vi "Base marwan_eleve.vi"() -> ()   [LabVIEW 2018]
uses:
  Global Humdidtiy 4.vi
  Global temperateurvi.vi
  Global  pressure.vi
  <vilib>/Instr/_visa.llb/VISA Configure Serial Port (Instr).vi
  <vilib>/express/express arith-compare/Formula/XNode/ExpressFormulaBlockNode.xnode
panel:
  out "Waveform Humidity 2":dbl(graph)
  out "Waveform Pressure 2":dbl(graph)
  out "Waveform temperateur  2":dbl(graph)
  out "Humidity 2":dbl
  out "Pressure 2":dbl
  out "Temperateur 2":dbl
  out "Chaîne 2":string
  out "Kelvin":dbl
  out "Fahrenheit":dbl
  in  "Pause":bool
  out "Moyen":dbl
  out "Moyen":dbl
  out "Moyen":dbl
  out "MAX":dbl
  out "MIN":dbl
  out "MIN":dbl
  out "MAX":dbl
  out "MIN":dbl
  out "MAX":dbl
  out "Waveform Humidity":dbl(graph)
  out "Waveform Pressure":dbl(graph)
  out "Waveform temperateur":dbl(graph)
  out "Humidity":dbl
  out "Pressure":dbl
  out "Temperateur":dbl
  out "Chaîne":string
  in  "stop":bool
  in  "Nom de ressource VISA":refnum<visa-resource-name>
  # "1. Brancher la carte Arduino sur un port USB\n2. Choisir le port COM de la carte dans la liste déroulante \"Nom de ressource VISA\"\n3. Lancer le programme"
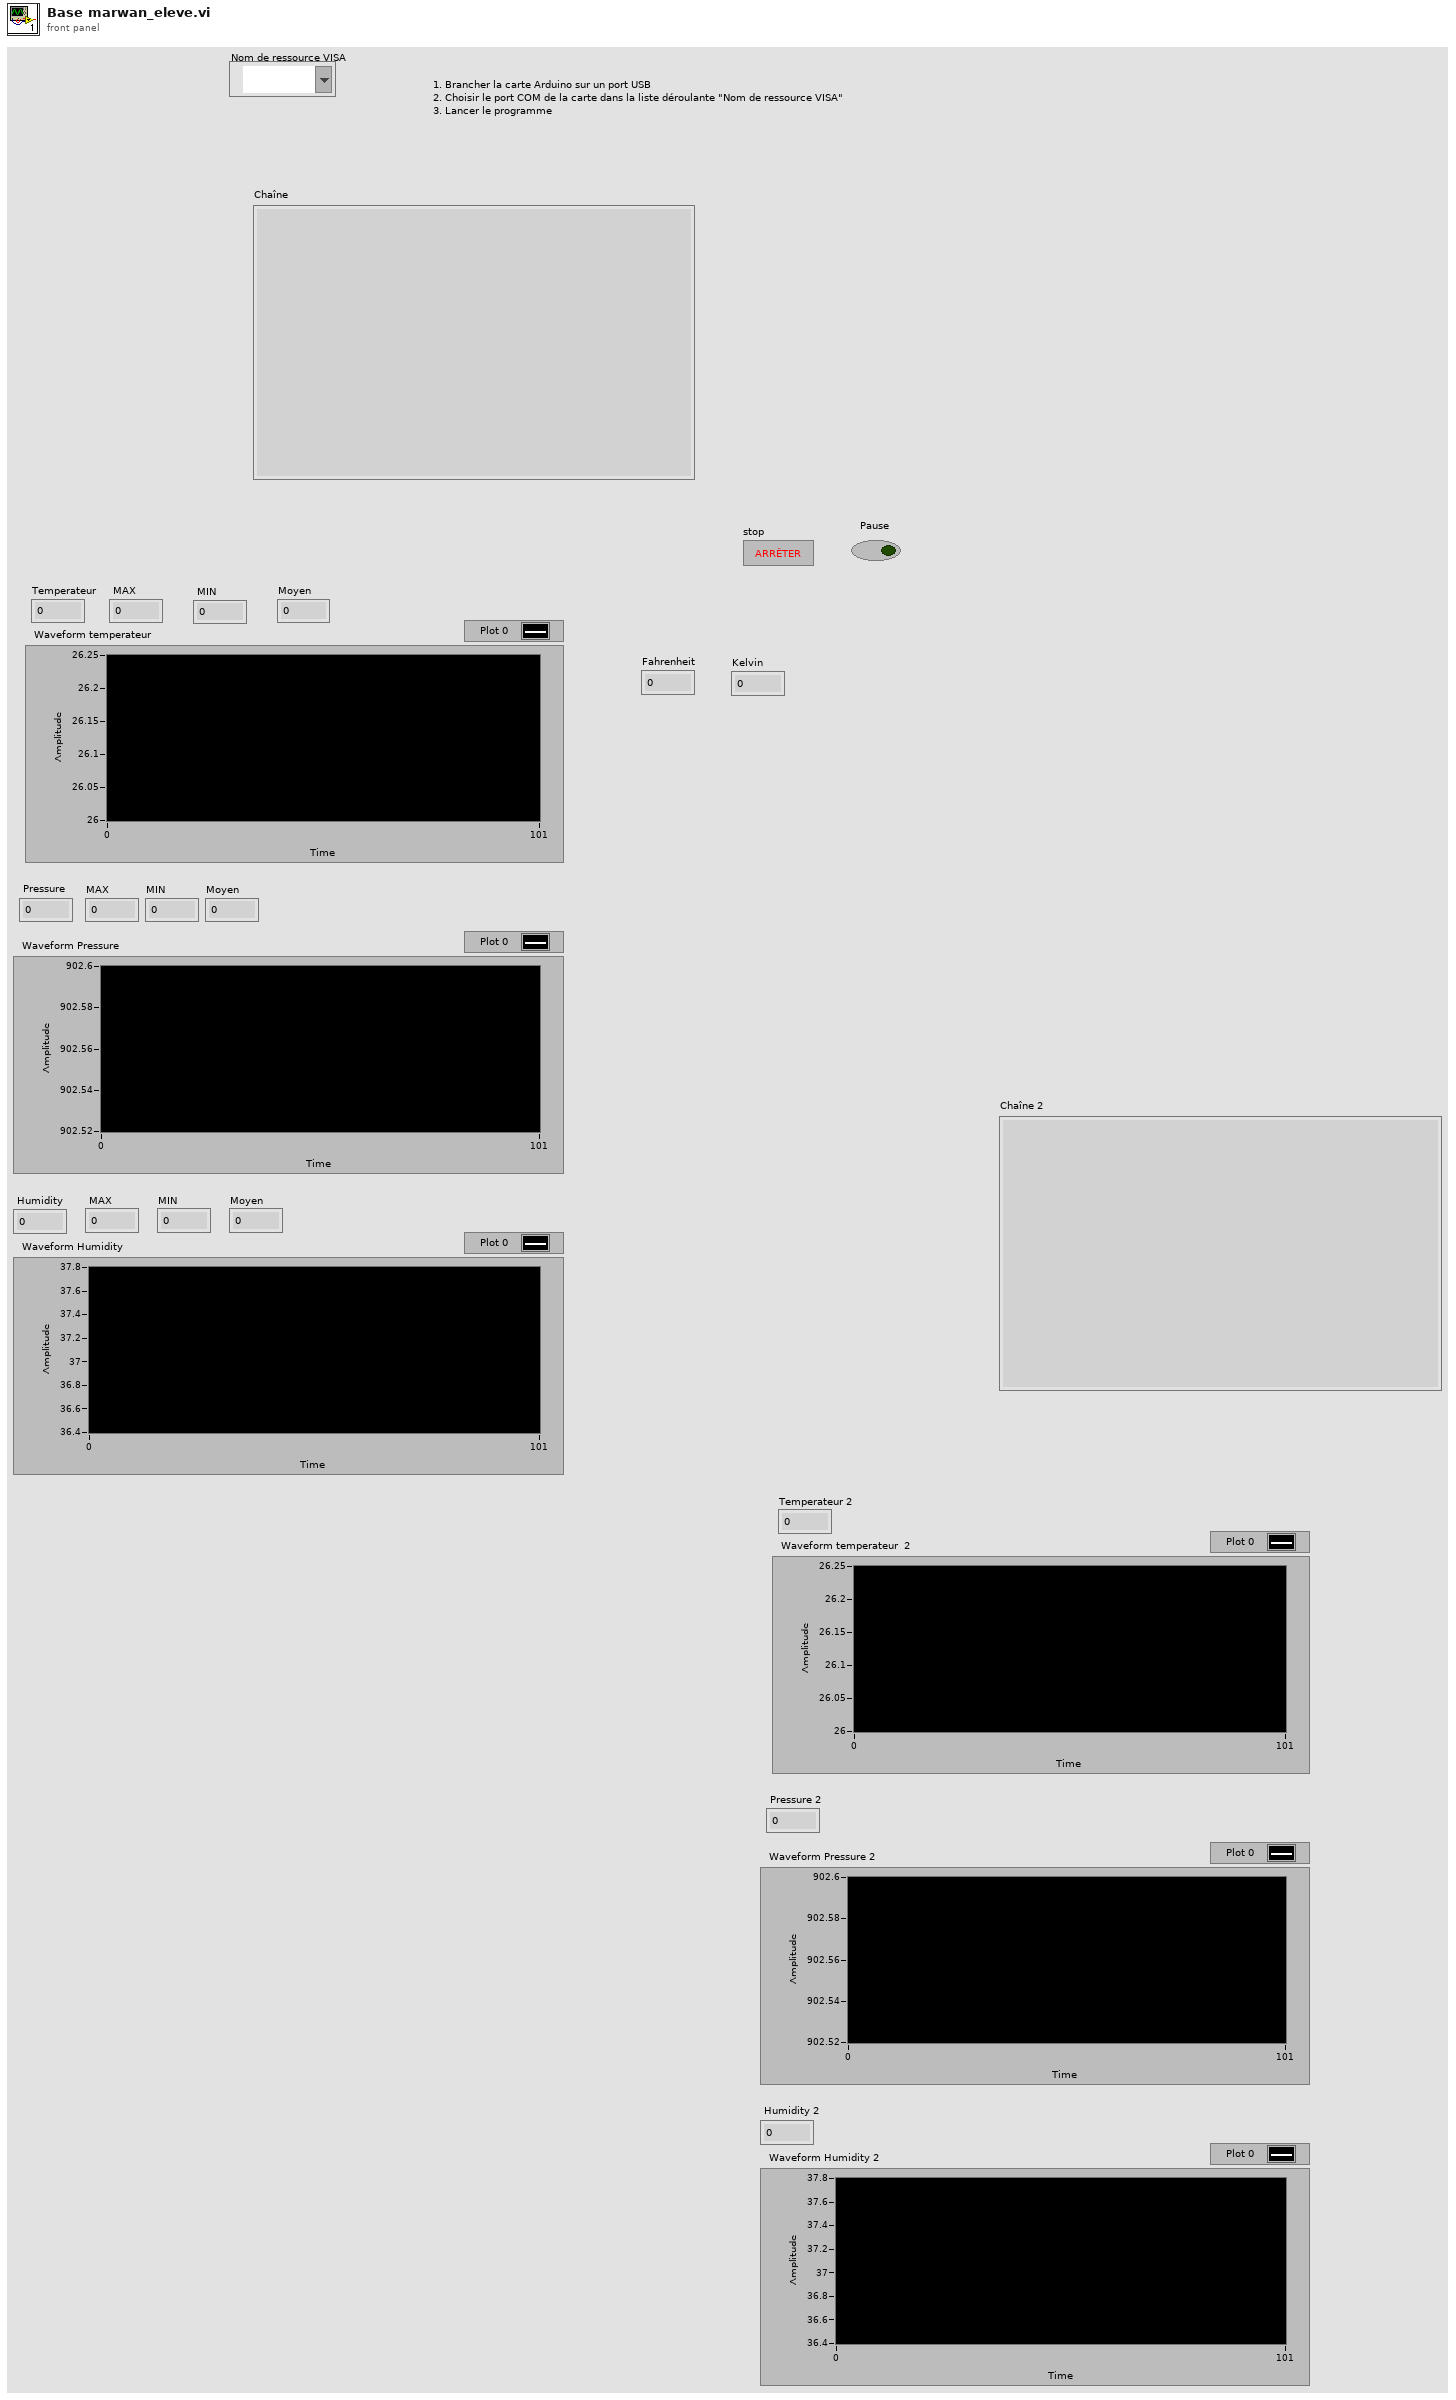
[diagram p1: front panel]
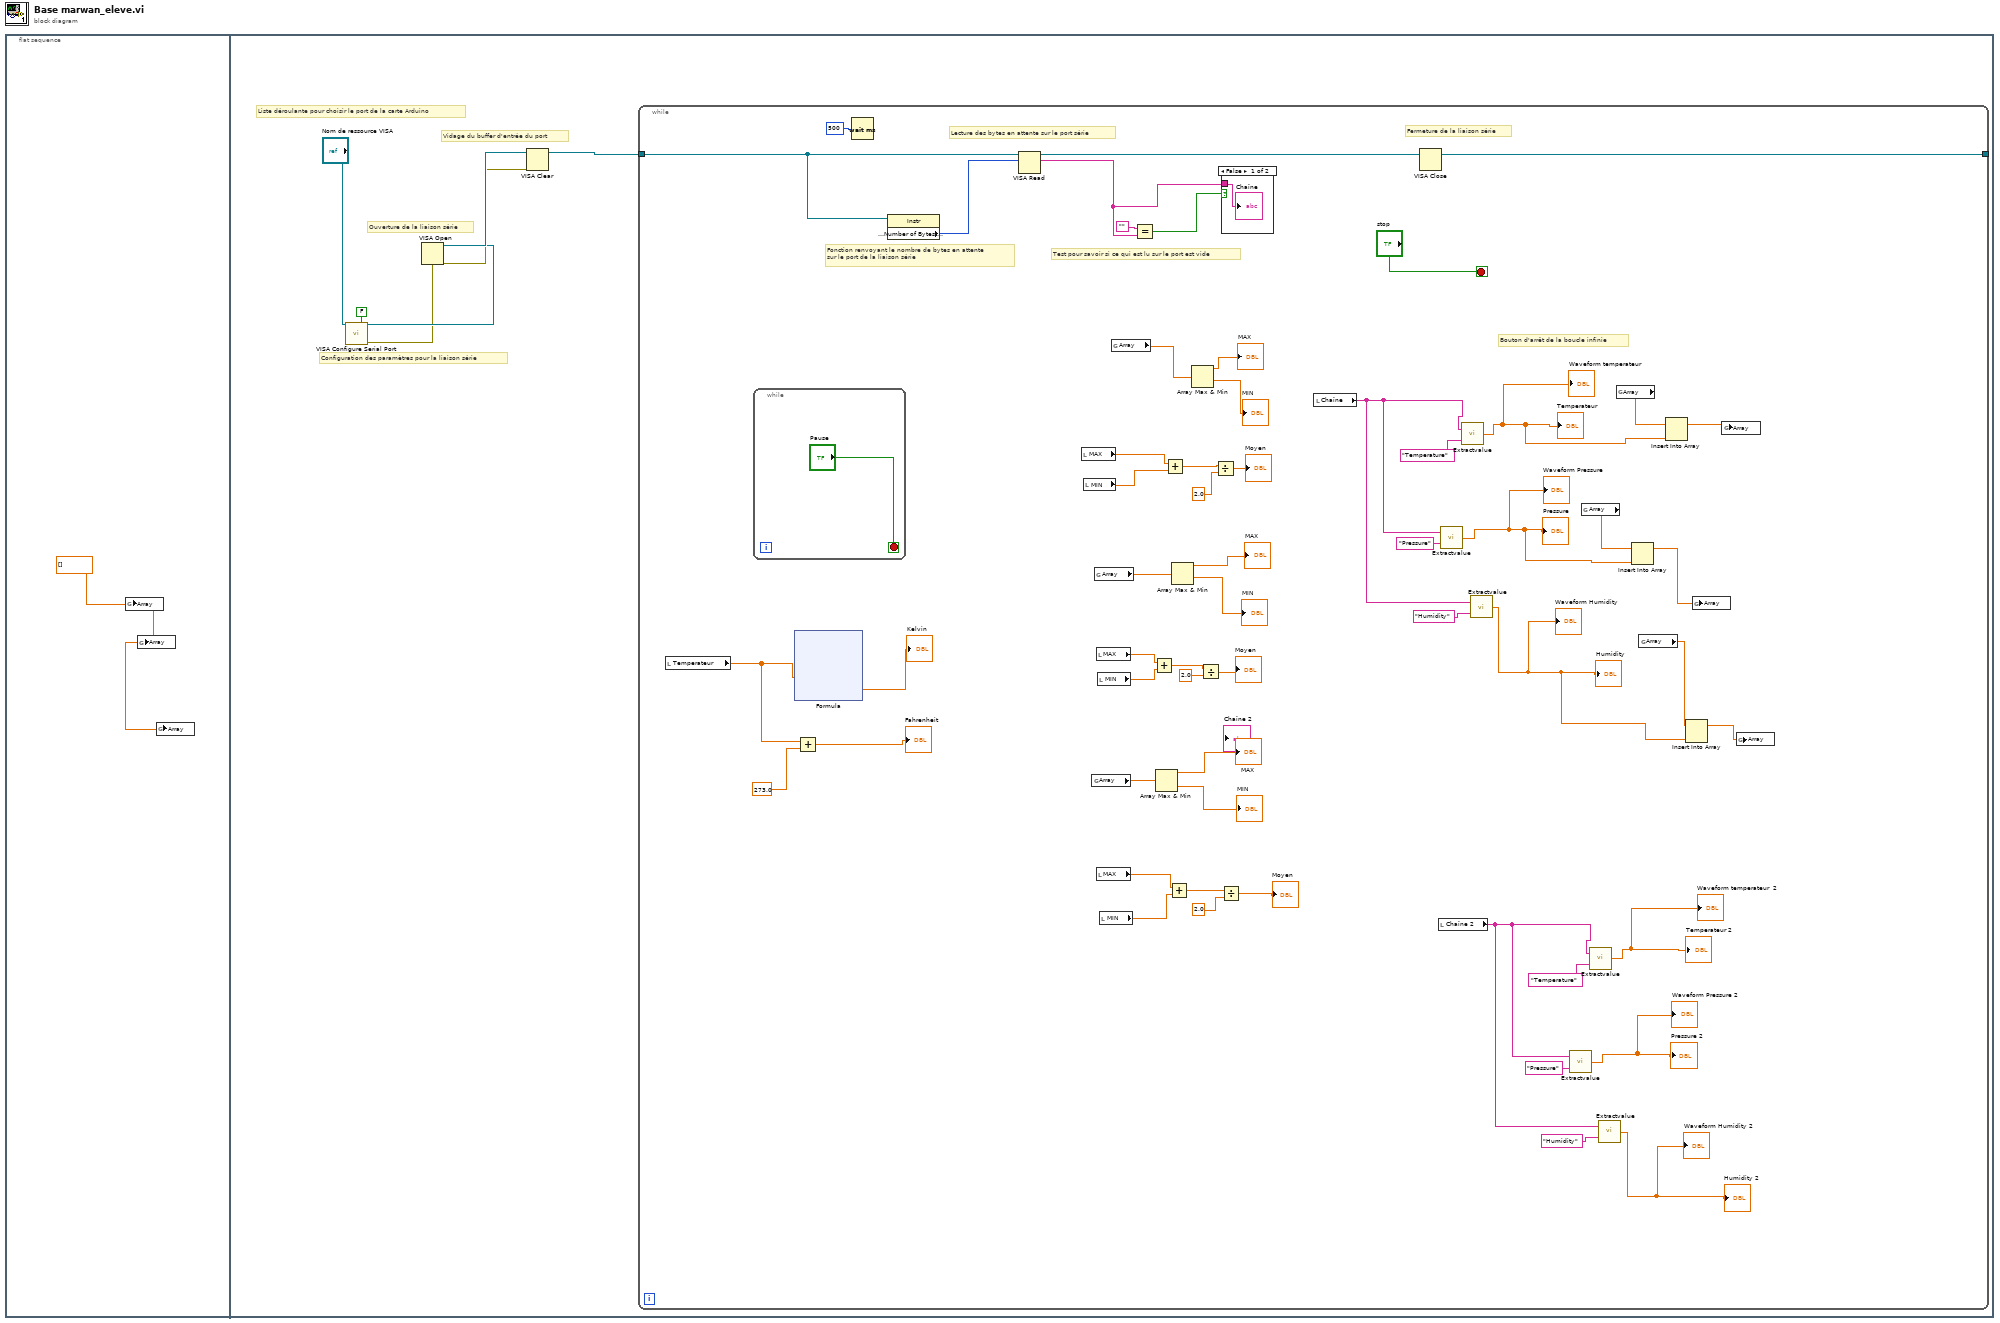
[diagram p0: block diagram]
diagram:
  n1 = flat-sequence {
    frame #0 {
      w1 = dbl[] []
      n2 = global write "Global  pressure.vi" "Array"(w1) -> ()
      n3 = global write "Global temperateurvi.vi" "Array"(w1) -> ()
      n4 = global write "Global Humdidtiy 4.vi" "Array"(w1) -> ()
    }
    frame #1 {
      # "Vidage du buffer d'entrée du port"
      # "Ouverture de la liaison série"
      # "Configuration des paramètres pour la liaison série"
      # "Liste déroulante pour choisir le port de la carte Arduino"
      # "Fermeture de la liaison série"
      n5 = call-poly "VISA Configure Serial Port"("VISA resource name"="Nom de ressource VISA", "Enable Termination\nChar (T)"=FALSE ("Enable Termination\nChar (T)")) -> ("VISA resource name out"=w6:refnum<visa-resource-name>, "error out"=w4:errorcluster)  [unwired: 12 in]
      n6 = VISA Open(error in (no error)=w4, VISA resource name=w6) -> (VISA resource name=w8:refnum<visa-resource-name>, error out=w3:errorcluster)  [unwired: 3 in]
      n7 = VISA Clear(VISA resource name=w8, error in (no error)=w3) -> (VISA resource name out=w7:refnum<visa-resource-name>)  [unwired: 1 out]
      n8 = while {
        tunnel: w7 -> [w64]
        tunnel: [w62] -> w2
        stop <- "stop" stop-if-true
        # "Lecture des bytes en attente sur le port série"
        # "Fonction renvoyant le nombre de bytes en attente\nsur le port de la liaison série"
        # "Test pour savoir si ce qui est lu sur le port est vide"
        # "Bouton d'arrêt de la boucle infinie"
        n9 = local read "Temperateur"() -> (w18:dbl)
        n10 = while {
          stop <- "Pause" stop-if-true
        }
        n11 = xnode "Formula"("X1"=w18) -> ("Result"=→"Kelvin":dbl)  [unwired: 1 in, 1 out]
        n12 = Add(x=w18, y=273.0) -> (x+y=→"Fahrenheit":dbl)
        n13 = Wait (ms)(milliseconds to wait=u32 500 ("attente (ms)")) -> ()  [unwired: 1 out]
        n14 = property class="Instr"(reference=w64) -> ("Serial Settings:Number of Bytes at Serial Port"=w63:u32)  [unwired: 1 in, 2 out]
        n15 = VISA Read(VISA resource name=w64, byte count=w63) -> (VISA resource name out=w62:refnum<visa-resource-name>, read buffer=w58:string)  [unwired: 1 in, 2 out]
        n16 = local read "MAX"() -> (w35:dbl)
        n17 = local read "MIN"() -> (w34:dbl)
        n18 = global read "Global Humdidtiy 4.vi" "Array"() -> (w38:dbl[])
        n19 = global read "Global  pressure.vi" "Array"() -> (w45:dbl[])
        n20 = local read "MAX"() -> (w30:dbl)
        n21 = local read "MAX"() -> (w25:dbl)
        n22 = local read "MIN"() -> (w29:dbl)
        n23 = local read "MIN"() -> (w24:dbl)
        n24 = global read "Global temperateurvi.vi" "Array"() -> (w50:dbl[])
        n25 = Equal?(x="", y=w58) -> (x = y?=w59:bool)
        n26 = Add(x=w30, y=w29) -> (x+y=w28:dbl)
        n27 = Array Max & Min(array=w38) -> (max value=→"MAX":dbl, min value=→"MIN":dbl)  [unwired: 2 out]
        n28 = Add(x=w35, y=w34) -> (x+y=w33:dbl)
        n29 = Add(x=w25, y=w24) -> (x+y=w23:dbl)
        n30 = Array Max & Min(array=w45) -> (max value=→"MAX":dbl, min value=→"MIN":dbl)  [unwired: 2 out]
        n31 = Array Max & Min(array=w50) -> (max value=→"MAX":dbl, min value=→"MIN":dbl)  [unwired: 2 out]
        n32 = Divide(x=w28, y=2.0) -> (x/y=→"Moyen":dbl)
        n33 = Divide(x=w33, y=2.0) -> (x/y=→"Moyen":dbl)
        n34 = Divide(x=w23, y=2.0) -> (x/y=→"Moyen":dbl)
        n35 = case shown="False" w59 {
          tunnel: w58 -> [w75 _]
          frame False {
            "Chaîne" <- w75
          }
          frame True {
          }
        }
        n36 = local read "Chaîne"() -> (w54:string)
        n37 = local read "Chaîne 2"() -> (w13:string)
        n38 = call "Extractvalue.vi"("Mesure"="Pressure", "Chaîne"=w54) -> ("Value"=w47:dbl)
        "Pressure" <- w47
        "Waveform Pressure" <- w47
        n39 = call "Extractvalue.vi"("Mesure"="Temperature", "Chaîne"=w54) -> ("Value"=w52:dbl)
        "Temperateur" <- w52
        "Waveform temperateur" <- w52
        n40 = call "Extractvalue.vi"("Mesure"="Humidity", "Chaîne"=w54) -> ("Value"=w41:dbl)
        "Humidity" <- w41
        "Waveform Humidity" <- w41
        n41 = call "Extractvalue.vi"("Mesure"="Pressure", "Chaîne"=w13) -> ("Value"=→"Pressure 2" →"Waveform Pressure 2":dbl)
        n42 = global read "Global  pressure.vi" "Array"() -> (w42:dbl[])
        n43 = call "Extractvalue.vi"("Mesure"="Temperature", "Chaîne"=w13) -> ("Value"=→"Temperateur 2" →"Waveform temperateur  2":dbl)
        n44 = call "Extractvalue.vi"("Mesure"="Humidity", "Chaîne"=w13) -> ("Value"=→"Humidity 2" →"Waveform Humidity 2":dbl)
        n45 = global read "Global temperateurvi.vi" "Array"() -> (w53:dbl[])
        n46 = Insert Into Array(array=w42, new element=w47) -> (w46:dbl[])  [unwired: 1 in]
        n47 = global read "Global Humdidtiy 4.vi" "Array"() -> (w40:dbl[])
        n48 = Insert Into Array(array=w53, new element=w52) -> (w51:dbl[])  [unwired: 1 in]
        n49 = Insert Into Array(array=w40, new element=w41) -> (w39:dbl[])  [unwired: 1 in]
        n50 = global write "Global  pressure.vi" "Array"(w46) -> ()
        n51 = global write "Global temperateurvi.vi" "Array"(w51) -> ()
        n52 = global write "Global Humdidtiy 4.vi" "Array"(w39) -> ()
      }
      n53 = VISA Close(VISA resource name=w2) -> ()  [unwired: 1 in, 1 out]
    }
  }
